vi "Highlight Leader.vi"(8 "error in (no error)":errorcluster, 11 "Controller in":refnum<class "Controller.lvclass">) -> (0 "error out":errorcluster, 3 "Controller out":refnum<class "Controller.lvclass">)   [LabVIEW 2023, in "Controller.lvlib" / "Controller.lvclass"]
uses:
  Controller.lvclass
  C:/Program Files/National Instruments/LabVIEW 2024/vi.lib/ActorFramework/Actor/Actor.lvclass
  <vilib>/ActorFramework/Actor/Actor.lvclass/Actor.ctl
  <vilib>/ActorFramework/Message Enqueuer/Message Enqueuer.lvclass/Message Enqueuer.ctl
  Controller.lvclass/Controller.ctl
  Controller Messages/Question Prompt Display Msg/Question Prompt Display Msg.lvclass/Question Prompt Display Msg.ctl
  <vilib>/ActorFramework/Message Enqueuer/Init from Existing Queue.vi
  <vilib>/ActorFramework/Message Enqueuer/Enqueue.vi
  Controller Messages/Question Prompt Display Msg/Question Prompt Display Msg.lvclass
  C:/Program Files/National Instruments/LabVIEW 2024/vi.lib/ActorFramework/Message/Message.lvclass
  <vilib>/ActorFramework/Message Priority Queue/Priority Enqueue.vi
  <vilib>/ActorFramework/Message Enqueuer/Message Enqueuer.lvclass
  <vilib>/ActorFramework/Actor/Actor.lvclass
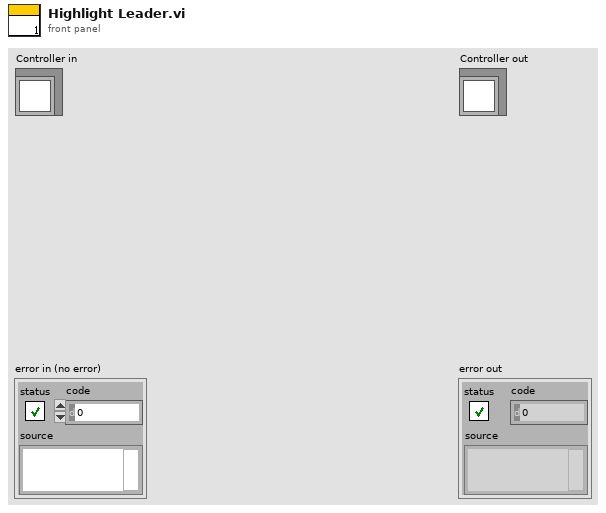
[diagram p1: front panel]
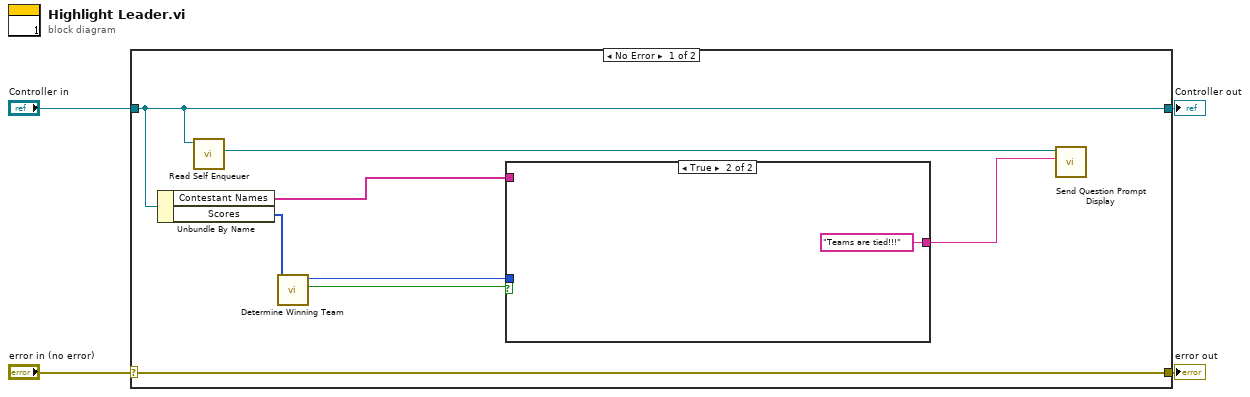
[diagram p0: block diagram]
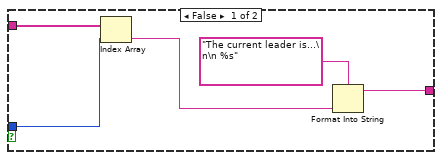
[diagram p2: hidden frame]
diagram:
  n1 = case shown="No Error" "error in (no error)" {
    selector: "error in (no error)" -> [w12 w20]
    tunnel: [w12 w20] -> w3
    tunnel: [w10 w19] -> w1
    tunnel: "Controller in" -> [w10 w19]
    frame No Error {
      n2 = Unbundle By Name(w10) -> ("Contestant Names"=w8:string[], "Scores"=w7:i32[])
      n3 = call <vilib>:"Read Self Enqueuer.vi"("Actor"=w10) -> ("Self Enqueuer"=w11:refnum<class "Message Enqueuer.lvclass">)  [unwired: 10 in]
      n4 = call "Determine Winning Team.vi"("Scores"=w7) -> ("Tie?"=w5:bool, "Index of Winner"=w6:i32)  [unwired: 9 in]
      n5 = case shown="True" w5 {
        tunnel: [w16 "Teams are tied!!!"] -> w9
        tunnel: w8 -> [w14 _]
        tunnel: w6 -> [w13 _]
        frame False {
          n6 = Index Array(array=w14, index=w13) -> (element=w15:string)
          n7 = Format Into String(format string="The current leader is...\n\n %s" ("Prompt"), w15) -> (resulting string=w16:string)  [unwired: 2 in, 1 out]
        }
        frame True {
        }
      }
      n8 = call "Send Question Prompt Display.vi"("Prompt"=w9, "Message Enqueuer"=w11) -> ()  [unwired: 8 in, 2 out]
    }
    frame Error {
    }
  }
  "error out" <- w3
  "Controller out" <- w1
